vi "LCR_TrimOC.vi"(8 "error in (no error)":errorcluster, 11 "HP4263B in":refnum<class "HP4263B.lvclass">) -> (0 "error out":errorcluster, 3 "HP4263B out":refnum<class "HP4263B.lvclass">)   [LabVIEW 2013, in "HP4263B.lvclass"]
uses:
  HP4263B.lvclass
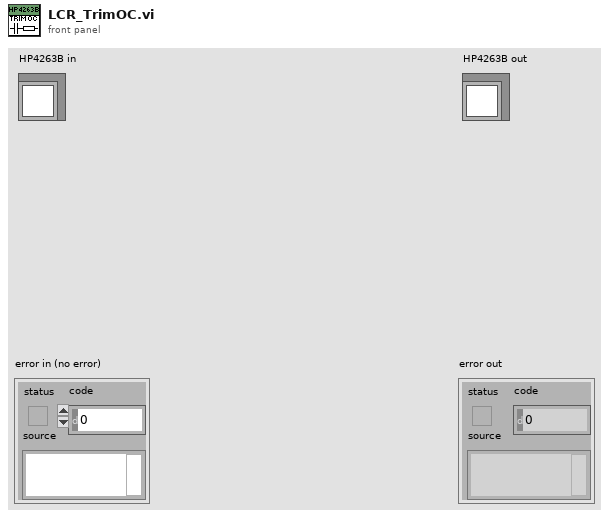
[diagram p1: front panel]
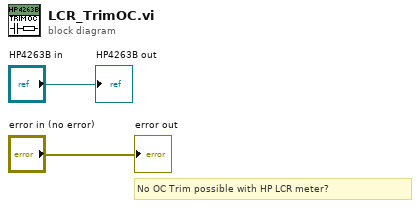
[diagram p0: block diagram]
diagram:
  # "No OC Trim possible with HP LCR meter?"
  "error out" <- "error in (no error)"
  "HP4263B out" <- "HP4263B in"
